vi "GUNSC_parse_rearrange.vi"(8 "error in (no error)":errorcluster, 10 "arguments":string) -> (0 "error out":errorcluster, 1 "func 3":string, 2 "func 2":string, 3 "func1":string, 4 "name2":string, 5 "name3":string, 6 "name1":string)   [LabVIEW 2016]
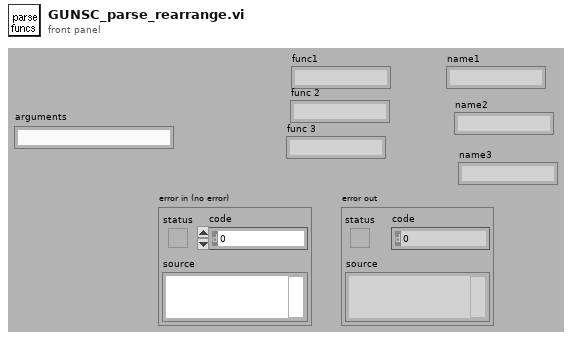
[diagram p1: front panel]
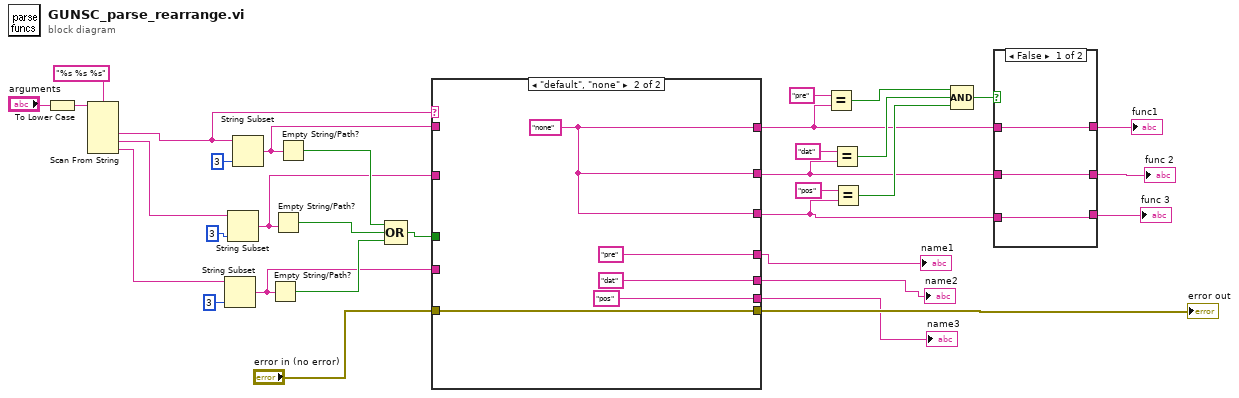
[diagram p0: block diagram]
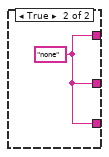
[diagram p2: hidden frame]
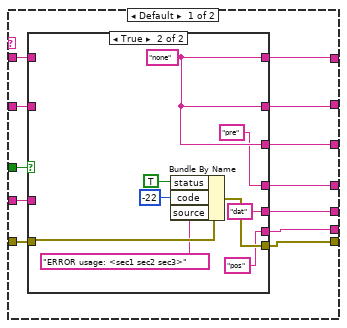
[diagram p3: hidden frame]
diagram:
  n1 = To Lower Case(string="arguments") -> (all lower case string=w31:string)
  n2 = Scan From String(format string="%s %s %s", input string=w31) -> (output 1=w23:string, output 2=w28:string, output 3=w27:string)  [unwired: 2 in, 6 out]
  n3 = String Subset(string=w27, length (rest)=3 ("length (rest)")) -> (substring=w19:string)  [unwired: 1 out]
  n4 = String Subset(string=w28, length (rest)=3 ("length (rest)")) -> (substring=w20:string)  [unwired: 1 out]
  n5 = String Subset(string=w23, length (rest)=3 ("length (rest)")) -> (substring=w21:string)  [unwired: 1 out]
  n6 = Empty String/Path?(string/path=w19) -> (empty?=w24:bool)
  n7 = Empty String/Path?(string/path=w20) -> (empty?=w25:bool)
  n8 = Empty String/Path?(string/path=w21) -> (empty?=w26:bool)
  n9 = Compound Arithmetic op=OR(w26, w25, w24) -> (w22:bool)
  n10 = case shown="\"default\", \"none\"" w23 {
    tunnel: [w40 w64] -> w6
    tunnel: [w39 w64] -> w5
    tunnel: [w38 w64] -> w4
    tunnel: w22 -> [w46 _]
    tunnel: w21 -> [w45 _]
    tunnel: w20 -> [w44 _]
    tunnel: w19 -> [w43 _]
    tunnel: "error in (no error)" -> [w42 w63]
    tunnel: [w41 w63] -> w17
    tunnel: [w37 "pre" ("x")] -> w3
    tunnel: [w36 "dat" ("x")] -> w2
    tunnel: [w35 "pos" ("x")] -> w1
    frame Default {
      n11 = case shown="True" w46 {
        tunnel: w45 -> [w49 _]
        tunnel: [w49 w59] -> w40
        tunnel: w44 -> [w48 _]
        tunnel: [w48 w59] -> w39
        tunnel: w43 -> [w47 _]
        tunnel: [w47 w59] -> w38
        tunnel: w42 -> [w50 w57]
        tunnel: [w50 w56] -> w41
        tunnel: [w49 "pre"] -> w37
        tunnel: [w48 "dat"] -> w36
        tunnel: [w47 "pos"] -> w35
        frame False {
        }
        frame True {
          w59 = "none"
          n12 = Bundle By Name(cluster=w57, "status"=TRUE, "code"=-22, "source"="ERROR usage: <sec1 sec2 sec3>") -> (w56:errorcluster)
        }
      }
    }
    frame "default", "none" {
      w64 = "none" ("func1")
    }
  }
  "error out" <- w17
  "name1" <- w3
  "name2" <- w2
  "name3" <- w1
  n13 = Equal?(x="pre", y=w6) -> (x = y?=w13:bool)
  n14 = Equal?(x="dat", y=w5) -> (x = y?=w12:bool)
  n15 = Equal?(x="pos", y=w4) -> (x = y?=w11:bool)
  n16 = Compound Arithmetic op=AND(w13, w12, w11) -> (w10:bool)
  n17 = case shown="False" w10 {
    tunnel: [w67 w68] -> w9
    tunnel: [w66 w68] -> w8
    tunnel: [w65 w68] -> w7
    tunnel: w6 -> [w67 _]
    tunnel: w5 -> [w66 _]
    tunnel: w4 -> [w65 _]
    frame False {
    }
    frame True {
      w68 = "none" ("func1")
    }
  }
  "func1" <- w9
  "func 2" <- w8
  "func 3" <- w7
